vi "URAPI_SystemCall.vi"(0 "Variable for reply":string="variable", 3 "URAPI Script":T1={"Script"="DIO[13] = 0\n", "Whiles"=[], "Ifs"=[], "Supress Err"=TRUE, "Errors"=""}, 4 "System call in":string="13,2") -> (2 "Variable Out":string="variable", 5 "URAPI Script":T1={"Script"="DIO[13] = 0\nSYSTEM 13,2\n", "Whiles"=[], "Ifs"=[], "Supress Err"=TRUE, "Errors"=""})   [LabVIEW 2012]
doc: "Calls customized system call on \"System call in\" and assigns \"variable for reply\" within the function"
uses:
  <userlib>/BotSpeak/VIs/Direct/URAPI_Control.ctl
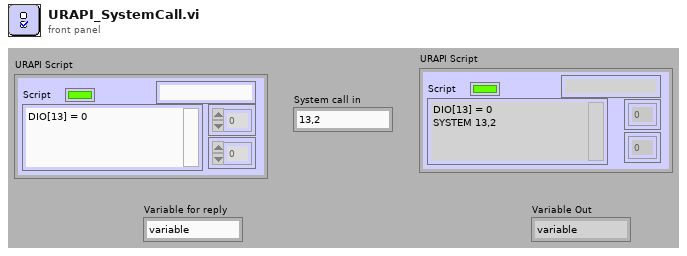
[diagram p1: front panel]
types:
  T1 = typedef "URAPI_Control.ctl" = cluster{"Script":string, "Whiles":u8[], "Ifs":u8[], "Supress Err":bool, "Errors":string}
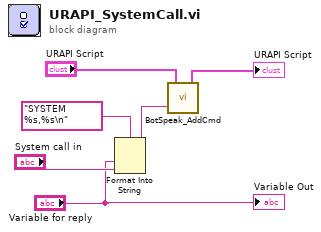
[diagram p0: block diagram]
diagram:
  n1 = Format Into String(format string="SYSTEM %s,%s\n" ("string"), "Variable for reply", "System call in") -> (resulting string=w3:string)  [unwired: 2 in, 1 out]
  n2 = call <userlib>:"BotSpeak_AddCmd.vi"("String"=w3, "URAPI Script"="URAPI Script") -> ("URAPI Script out"=→"URAPI Script":T1)  [unwired: 1 in]
  "Variable Out" <- "Variable for reply"
